vi "OutPutMAP.vi"(7 "Outputs":i32[](array[numeric]), 8 "error in (no error)":errorcluster, 9 "Variables State in":T1, 10 "HW CTRL Data":T2, 11 "I/O Map In":T4) -> (0 "error out":errorcluster, 1 "DO Status":i32[](array[numeric]), 2 "DO Out":bool[][](array[boolean]))   [LabVIEW 2014]
doc: "Mapea las salidas y chequea la Ecuación lógica de seguridad."
uses:
  TypeDefs/HW InOut MAP.ctl
  TypeDefs/LogicParsedExpression.ctl
  TypeDefs/HW CTRL Data.ctl
  TypeDefs/HW Variables State.ctl
  SeqLoop.lvlib
panel:
  in  "Logical Parsed Expression":T3
  out "I/O Map Out":T4
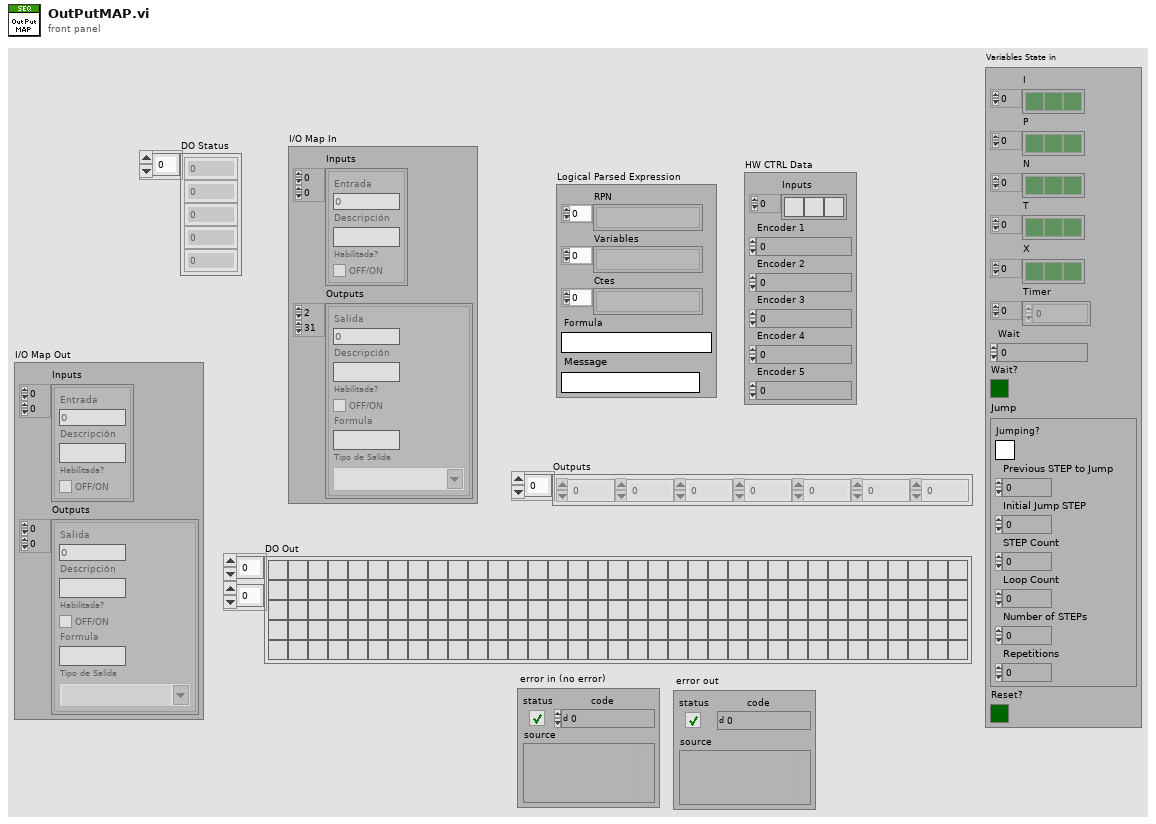
[diagram p1: front panel]
types:
  T1 = typedef "SeqLoop.lvlib/HW Variables State.ctl" = cluster{"I":bool[], "P":bool[], "N":bool[], "T":bool[], "X":bool[], "Timer":u32[], "Wait":u32, "Wait?":bool, "Jump":cluster{"Jumping?":bool, "Previous STEP to Jump":u32, "Initial Jump STEP":u32, "STEP Count":u32, "Loop Count":u32, "Number of STEPs":u32, "Repetitions":u32}, "Reset?":bool}
  T2 = typedef "SeqLoop.lvlib/HW CTRL Data.ctl" = cluster{"Inputs":bool[], "Encoder 1":sgl, "Encoder 2":sgl, "Encoder 3":sgl, "Encoder 4":sgl, "Encoder 5":sgl}
  T3 = typedef "SeqLoop.lvlib/LogicParsedExpression.ctl" = cluster{"RPN ":string[], "Variables":string[], "Ctes":string[], "Formula":string, "Message":string}
  T4 = typedef "SeqLoop.lvlib/HW InOut MAP.ctl" = cluster{"Inputs":cluster{"Entrada":i32, "Descripción":string, "Habilitada?":bool}[][], "Outputs":cluster{"Salida":i32, "Descripción":string, "Habilitada?":bool, "Formula":string, "Tipo de Salida":string}[][]}
  T5 = cluster{"Salida":i32, "Descripción":string, "Habilitada?":bool, "Formula":string, "Tipo de Salida":string}[][]
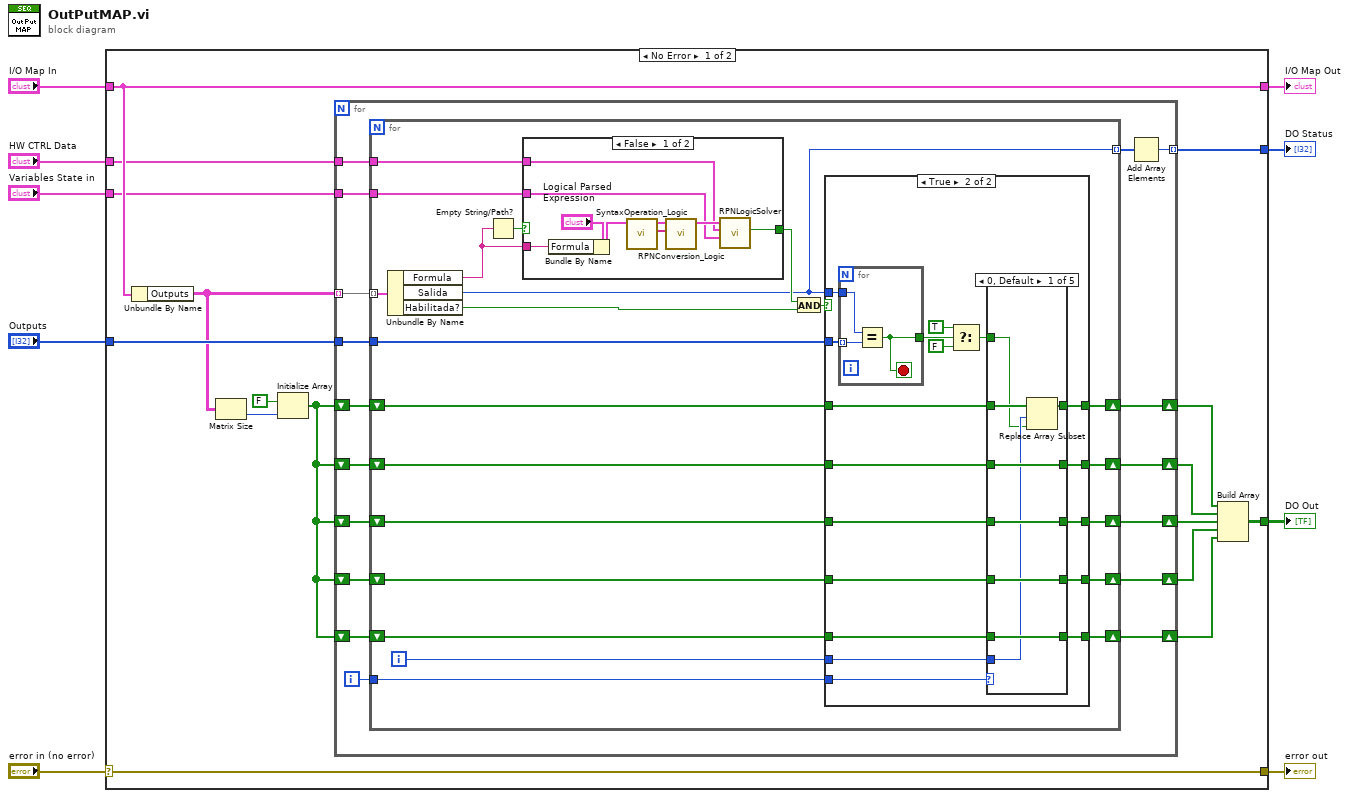
[diagram p0: block diagram]
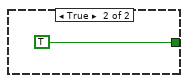
[diagram p2: hidden frame]
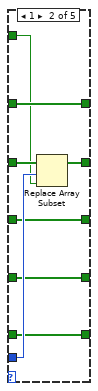
[diagram p4: hidden frame]
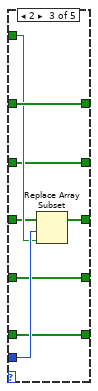
[diagram p5: hidden frame]
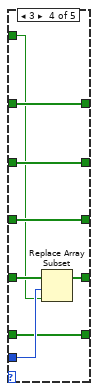
[diagram p6: hidden frame]
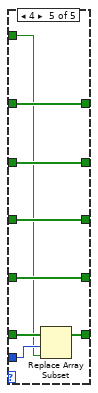
[diagram p7: hidden frame]
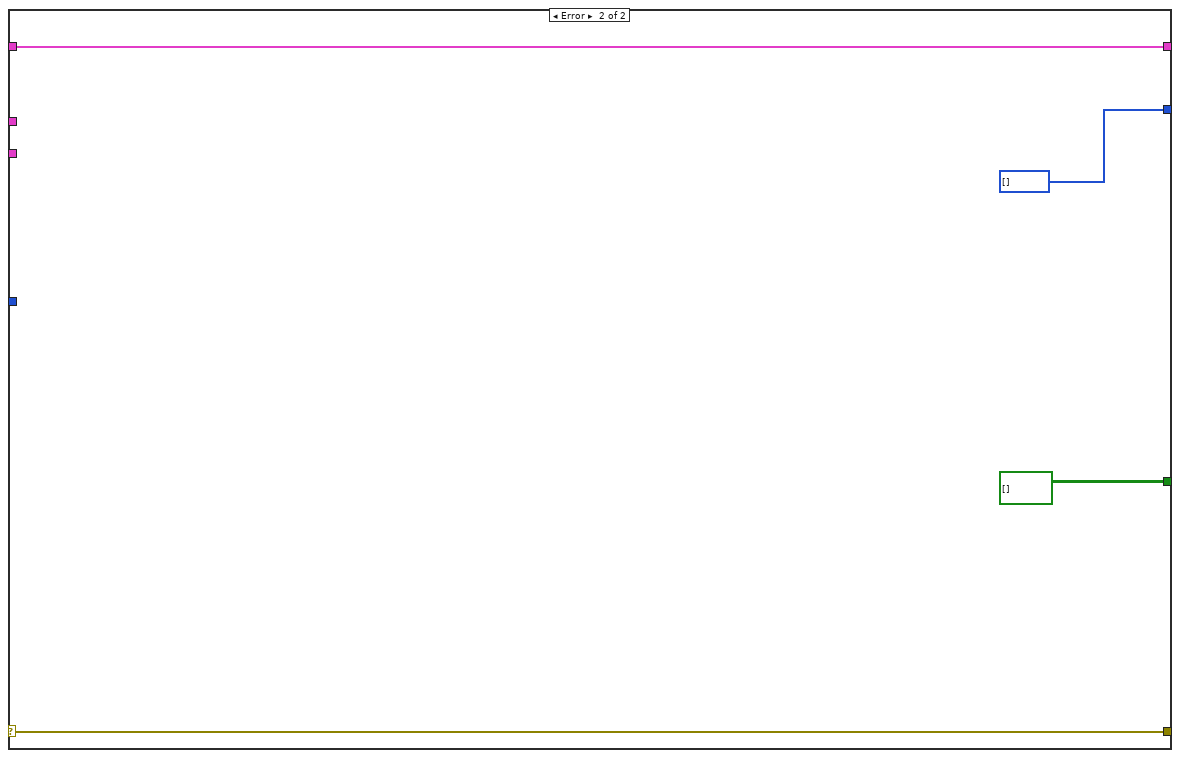
[diagram p8: hidden frame]
diagram:
  n1 = case shown="No Error" "error in (no error)" {
    selector: "error in (no error)" -> [w23 w143]
    tunnel: [w23 w143] -> w3
    tunnel: "I/O Map In" -> [w25 w144]
    tunnel: [w25 w144] -> w7
    tunnel: "Outputs" -> [w24 _]
    tunnel: [w13 bool[][] []] -> w5
    tunnel: [w12 i32[] []] -> w4
    tunnel: "HW CTRL Data" -> [w11 _]
    tunnel: "Variables State in" -> [w10 _]
    frame No Error {
      n2 = Unbundle By Name(w25) -> ("Outputs"=w17:T5)
      n3 = Matrix Size(0:w17) -> (2:w15:i32)  [unwired: 1 out]
      n4 = Initialize Array(FALSE ("f"), w15) -> (w14:bool[])
      n5 = for {
        tunnel: w17 -> [w42] mode=indexing
        tunnel: w24 -> [w41]
        shift-right: [w33] -> w22
        shift-left: w14 -> [w40]
        shift-right: [w32] -> w21
        shift-left: w14 -> [w39]
        shift-right: [w31] -> w20
        shift-left: w14 -> [w38]
        shift-right: [w34] -> w19
        shift-left: w14 -> [w37]
        shift-right: [w35] -> w18
        shift-left: w14 -> [w36]
        tunnel: [w28] -> w12 mode=indexing
        tunnel: w11 -> [w27]
        tunnel: w10 -> [w26]
        i -> [w30]
        n6 = for {
          tunnel: w42 -> [w64] mode=indexing
          tunnel: w41 -> [w63]
          tunnel: w30 -> [w62]
          shift-right: [w53] -> w33
          shift-left: w40 -> [w56]
          shift-right: [w52] -> w32
          shift-left: w39 -> [w55]
          shift-right: [w51] -> w31
          shift-left: w38 -> [w54]
          shift-right: [w57] -> w34
          shift-left: w37 -> [w58]
          shift-right: [w59] -> w35
          shift-left: w36 -> [w60]
          tunnel: [w45] -> w29 mode=indexing
          tunnel: w27 -> [w47]
          tunnel: w26 -> [w46]
          i -> [w61]
          n7 = Unbundle By Name(w64) -> ("Formula"=w43:string, "Salida"=w45:i32, "Habilitada?"=w49:bool)
          n8 = Empty String/Path?(string/path=w43) -> (empty?=w44:bool)
          n9 = case shown="False" w44 {
            tunnel: [w68 TRUE ("Logic Result")] -> w50
            tunnel: w47 -> [w67 _]
            tunnel: w46 -> [w66 _]
            tunnel: w43 -> [w65 _]
            frame False {
              n10 = Bundle By Name(cluster="Logical Parsed Expression", "Formula"=w65) -> (w69:T3)
              n11 = call "SyntaxOperation_Logic.vi"("Logical Parsed Expression"=w69) -> ("Token"=w72:string[], "Logical Parsed Expression Out"=w73:T3)  [unwired: 7 in, 2 out]
              n12 = call "RPNConversion_Logic.vi"("Token"=w72, "Logical Parsed Expression"=w73) -> ("Logical Parsed Expression Out"=w71:T3)  [unwired: 8 in, 1 out]
              n13 = call "RPNLogicSolver.vi"("Variables State in"=w66, "HW CTRL Data"=w67, "Logic Parsed Expression"=w71) -> ("Logic Result"=w68:bool)  [unwired: 6 in, 2 out]
            }
            frame True {
            }
          }
          n14 = And(x=w50, y=w49) -> (x .and. y?=w48:bool)
          n15 = case shown="True" w48 {
            tunnel: w45 -> [_ w89]
            tunnel: w63 -> [_ w90]
            tunnel: w62 -> [_ w97]
            tunnel: w61 -> [_ w96]
            tunnel: [w79 w80] -> w53
            tunnel: [w78 w81] -> w52
            tunnel: [w77 w82] -> w51
            tunnel: [w76 w83] -> w57
            tunnel: [w75 w84] -> w59
            tunnel: w60 -> [w75 w95]
            tunnel: w58 -> [w76 w94]
            tunnel: w54 -> [w77 w93]
            tunnel: w55 -> [w78 w92]
            tunnel: w56 -> [w79 w91]
            frame False {
            }
            frame True {
              n16 = for {
                tunnel: w90 -> [w99] mode=indexing
                tunnel: w89 -> [w100]
                tunnel: [w98] -> w86
                stop <- w98 stop-if-true
                n17 = Equal?(x=w100, y=w99) -> (x = y?=w98:bool)
              }
              n18 = Select(t=TRUE, s=w86, f=FALSE) -> (s? t:f=w85:bool)
              n19 = case shown="0, Default" w97 {
                tunnel: w96 -> [w102 w113 w123 w127 w134]
                tunnel: [w103 w116 w124 w132 w140] -> w80
                tunnel: [w106 w114 w119 w131 w135] -> w81
                tunnel: [w105 w111 w117 w130 w136] -> w82
                tunnel: [w107 w110 w121 w128 w137] -> w83
                tunnel: [w108 w109 w120 w125 w138] -> w84
                tunnel: w95 -> [w108 w109 w120 w125 w139]
                tunnel: w94 -> [w107 w110 w121 w129 w137]
                tunnel: w93 -> [w105 w111 w118 w130 w136]
                tunnel: w92 -> [w106 w115 w119 w131 w135]
                tunnel: w91 -> [w104 w116 w124 w132 w140]
                tunnel: w85 -> [w101 w112 w122 w126 w133]
                frame 0, Default {
                  n20 = Replace Array Subset(array=w104, new element=w101, index=w102) -> (w103:bool[])
                }
                frame 1 {
                  n21 = Replace Array Subset(array=w115, new element=w112, index=w113) -> (w114:bool[])
                }
                frame 2 {
                  n22 = Replace Array Subset(array=w118, new element=w122, index=w123) -> (w117:bool[])
                }
                frame 3 {
                  n23 = Replace Array Subset(array=w129, new element=w126, index=w127) -> (w128:bool[])
                }
                frame 4 {
                  n24 = Replace Array Subset(array=w139, new element=w133, index=w134) -> (w138:bool[])
                }
              }
            }
          }
        }
        n25 = Add Array Elements(numeric array=w29) -> (sum=w28:i32)
      }
      n26 = Build Array(w22, w21, w20, w19, w18) -> (w13:bool[][])
    }
    frame Error {
    }
  }
  "I/O Map Out" <- w7
  "error out" <- w3
  "DO Out" <- w5
  "DO Status" <- w4
